vi "WriteParameter.vi"(6 "TimeOut(500)":i32=500, 9 "test":dbl[](array[numeric])=[0.0, 1.0, 111111111111111.0, 1.0, 2.0, 1.0, 1.0, 10.0, 0.0, 0.0, 0.0, 0.0, 500.0, 250.0, 2.0, 2.0, 2.0, 2.0, 0.0, 0.0, 0.0], 11 "UnitParamiterCluster":T1={"External Diameter"=0.0, "Height"=0.0, "Range"=enum."1p", "DFmin"=0.00024, "Cap_num"=0.0, "F"=0, "BIN3+"=0.0, "BIN3- "=0.0, "BIN2+"=0.0, "BIN2-"=0.0, "BIN1+"=0.0, "BIN1-"=0.0, "Frequencies"=enum."120HZ", "DFmax"=0.00024, "Part_5"=0.0, "Part_6"=0.0, "Part_4"=5.0, "Part_8"=7.0, "Part_7"=4.0, "Par_2"=4.0, "part_1"=enum."DC", "Part_9"=9.0, "Part_18"=7.0, "Part_15"=3.0, "Part_13"=2.0, "Part_14"=5.0, "Part_16"=6.0, "Internal Diameter"=0.0, "Part_14 (IR Max)"=1000000000000000.0, "SCARA Place Offset"={"Buffer"={"X"=0.0, "Y"=0.0, "Z"=0.0}, "UNLD"={"X"=0.0, "Y"=0.0, "Z"=0.0}}} {"Part_14 (IR Max)" format="%#_6p"; "Part_6" format="%#_9g"; "DFmin" format="%#_9g"; "Cap_num" format="%#_9f"; "F" items=["mF", "uF", "nF", "pF"]}) -> (0 "HiokiErrout":errorcluster, 1 "ChromaErrOut":errorcluster, 3 "TVwriteOK":bool[](array[boolean]))   [LabVIEW 2016]
uses:
  TypeDef/Enum_ErrorType.ctl
  DISGradingMachine/SubPannel/PNType/TypeDef_PNData.ctl
  DISGradingMachine/sub/MachineParType/MachineParTypeSCARA PlaceOffset.ctl
  meter global.vi
  <vilib>/Instr/_visa.llb/VISA Configure Serial Port (Instr).vi
panel:
  out "read buffer":string
  out "TV1":T3
  # "TV參數修改中,請稍候......."
  # "尺寸資訊"
  # "max 3mm  0=1mm"
  # "大於 3.56mm=0"
  # "電性測試"
  # "%"
  # "%"
  # "%"
  # "%"
  # "%"
  # "%"
  # "IR 絕緣阻抗測試"
  # "V"
  # "sec"
  # "sec"
  # "sec"
  # "GΩ"
  # "Ω"
  # "TV   耐壓測試"
  # "sec"
  # "uA"
  # "sec"
  # "KV"
  # "sec"
  # "uA"
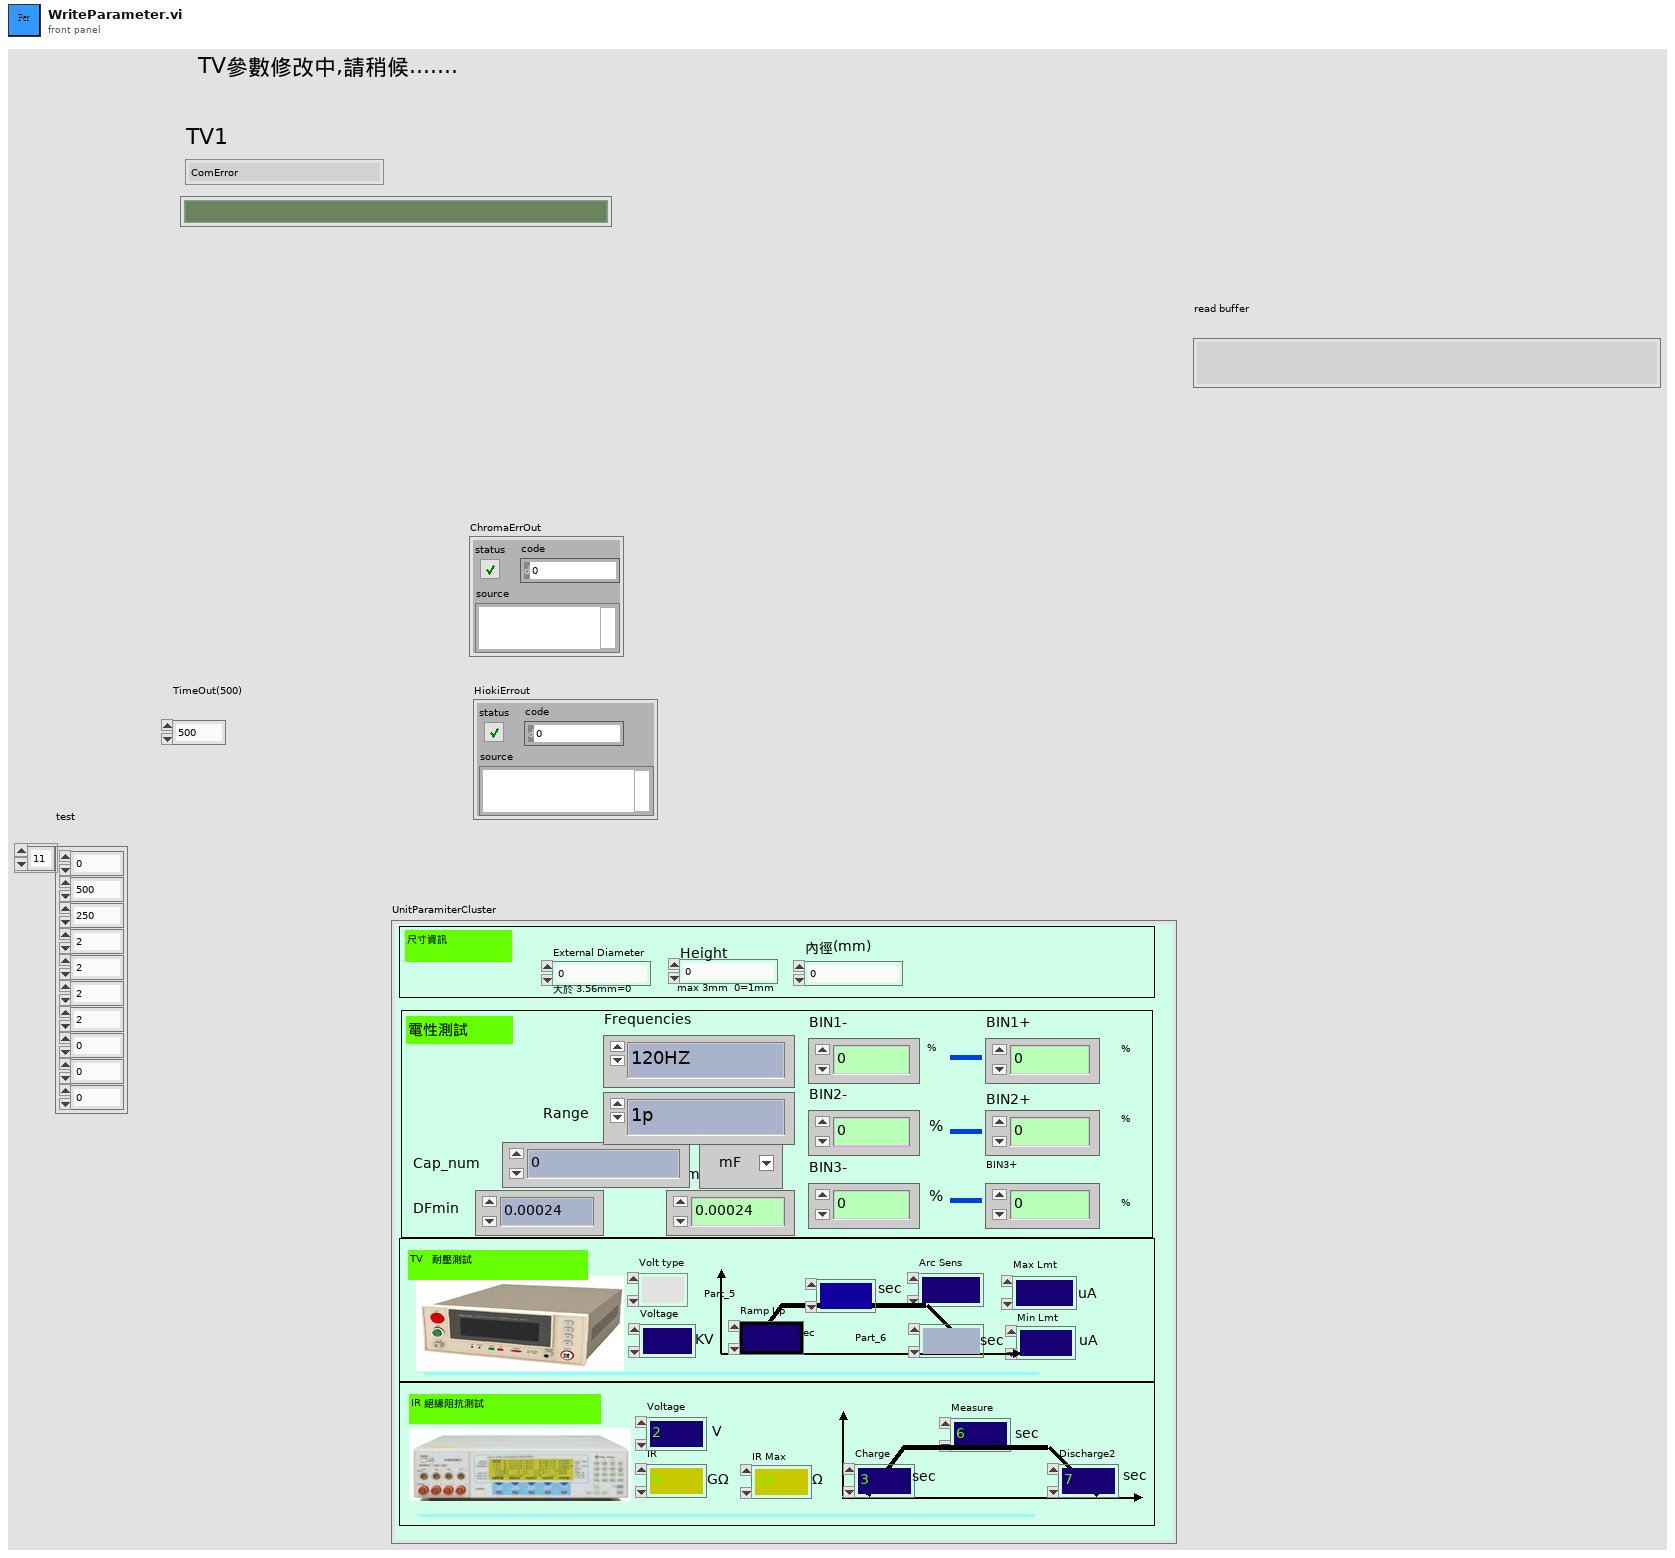
[diagram p1: front panel]
types:
  T1 = typedef "TypeDef_PNData.ctl" = cluster{"External Diameter":dbl, "Height":dbl, "Range":enum16{"1p", "2.2p", "4.7p", "10p", "22p", "47p", "100p", "220p", "470p", "1n", "2.2n", "4.7n", "10n", "22n", "47n", "100n", "220n", "470n", "1u", "2.2u", "4.7u", "10u", "22u", "47u", "100u", "220u", "470u", "1m", "AUTO", ""}, "DFmin":dbl, "Cap_num":dbl, "F":u16, "BIN3+":dbl, "BIN3- ":dbl, "BIN2+":dbl, "BIN2-":dbl, "BIN1+":dbl, "BIN1-":dbl, "Frequencies":enum16{"120HZ", "1K  HZ", "1M HZ"}, "DFmax":dbl, "Part_5":dbl, "Part_6":dbl, "Part_4":dbl, "Part_8":dbl, "Part_7":dbl, "Par_2":dbl, "part_1":enum16{"DC", "AC"}, "Part_9":dbl, "Part_18":dbl, "Part_15":dbl, "Part_13":dbl, "Part_14":dbl, "Part_16":dbl, "Internal Diameter":dbl, "Part_14 (IR Max)":dbl, "SCARA Place Offset":T2}
  T2 = typedef "MachineParTypeSCARA PlaceOffset.ctl" = cluster{"Buffer":cluster{"X":dbl, "Y":dbl, "Z":dbl}, "UNLD":cluster{"X":dbl, "Y":dbl, "Z":dbl}}
  T3 = typedef "Enum_ErrorType.ctl" = enum16{"ComError", "OK", "Command Error", "Parameter Error"}
  T4 = cluster{"Enum_mode":enum16{"AC", "DC", "IR"}, "StepIndex(1~10)":u8, "RampTime(100ms)":u16, "DwallTime(100ms)":u16, "TestTime(100ms)":u16, "Falltime(100ms)":u16, "HighLimit(100nA)":u32, "LowLimit(100nA)":u32, "ArcLimit(100nA)":u32, "InrushLimit(100nA)":u32, "Sorce(v)":u16}
  T5 = enum16{"RDT?", "IDN?", "SRT", "CBF", "SEQ?", "RMT", "SEQ", "PWS", "STP", "PWS?", "PWA", "CHS", ""}
  T6 = enum16{"RDT?", "IDN?", "SRT", "CBF", "SEQ?", "RMT", "SEQ", "PWS", "STP", "PWS?", "PWA"}
  T7 = cluster{"OFF:0/ON:1":i32, "Program Number(0~9)":i32, "DischargeTimeBeforeMeasurement":dbl, "ChargeTime":dbl, "Measuring Time":dbl, "DisCharge Time":dbl}
  T8 = cluster{"EnumFunnction":enum16{"IDN?", "test", "Stop", "Start", "Step Parameters", "Step Patameters?", "Preset Parameter", "Preset parameter?", "Offset Get/Off", "Offset?", "System Setting", "System Setting?", "KeyLock", "KeyLock?", "Initialize All Steps Parameter", "Remote/Local", "Result"}, "Hex_DA":u8, "Hex_Master":u8}
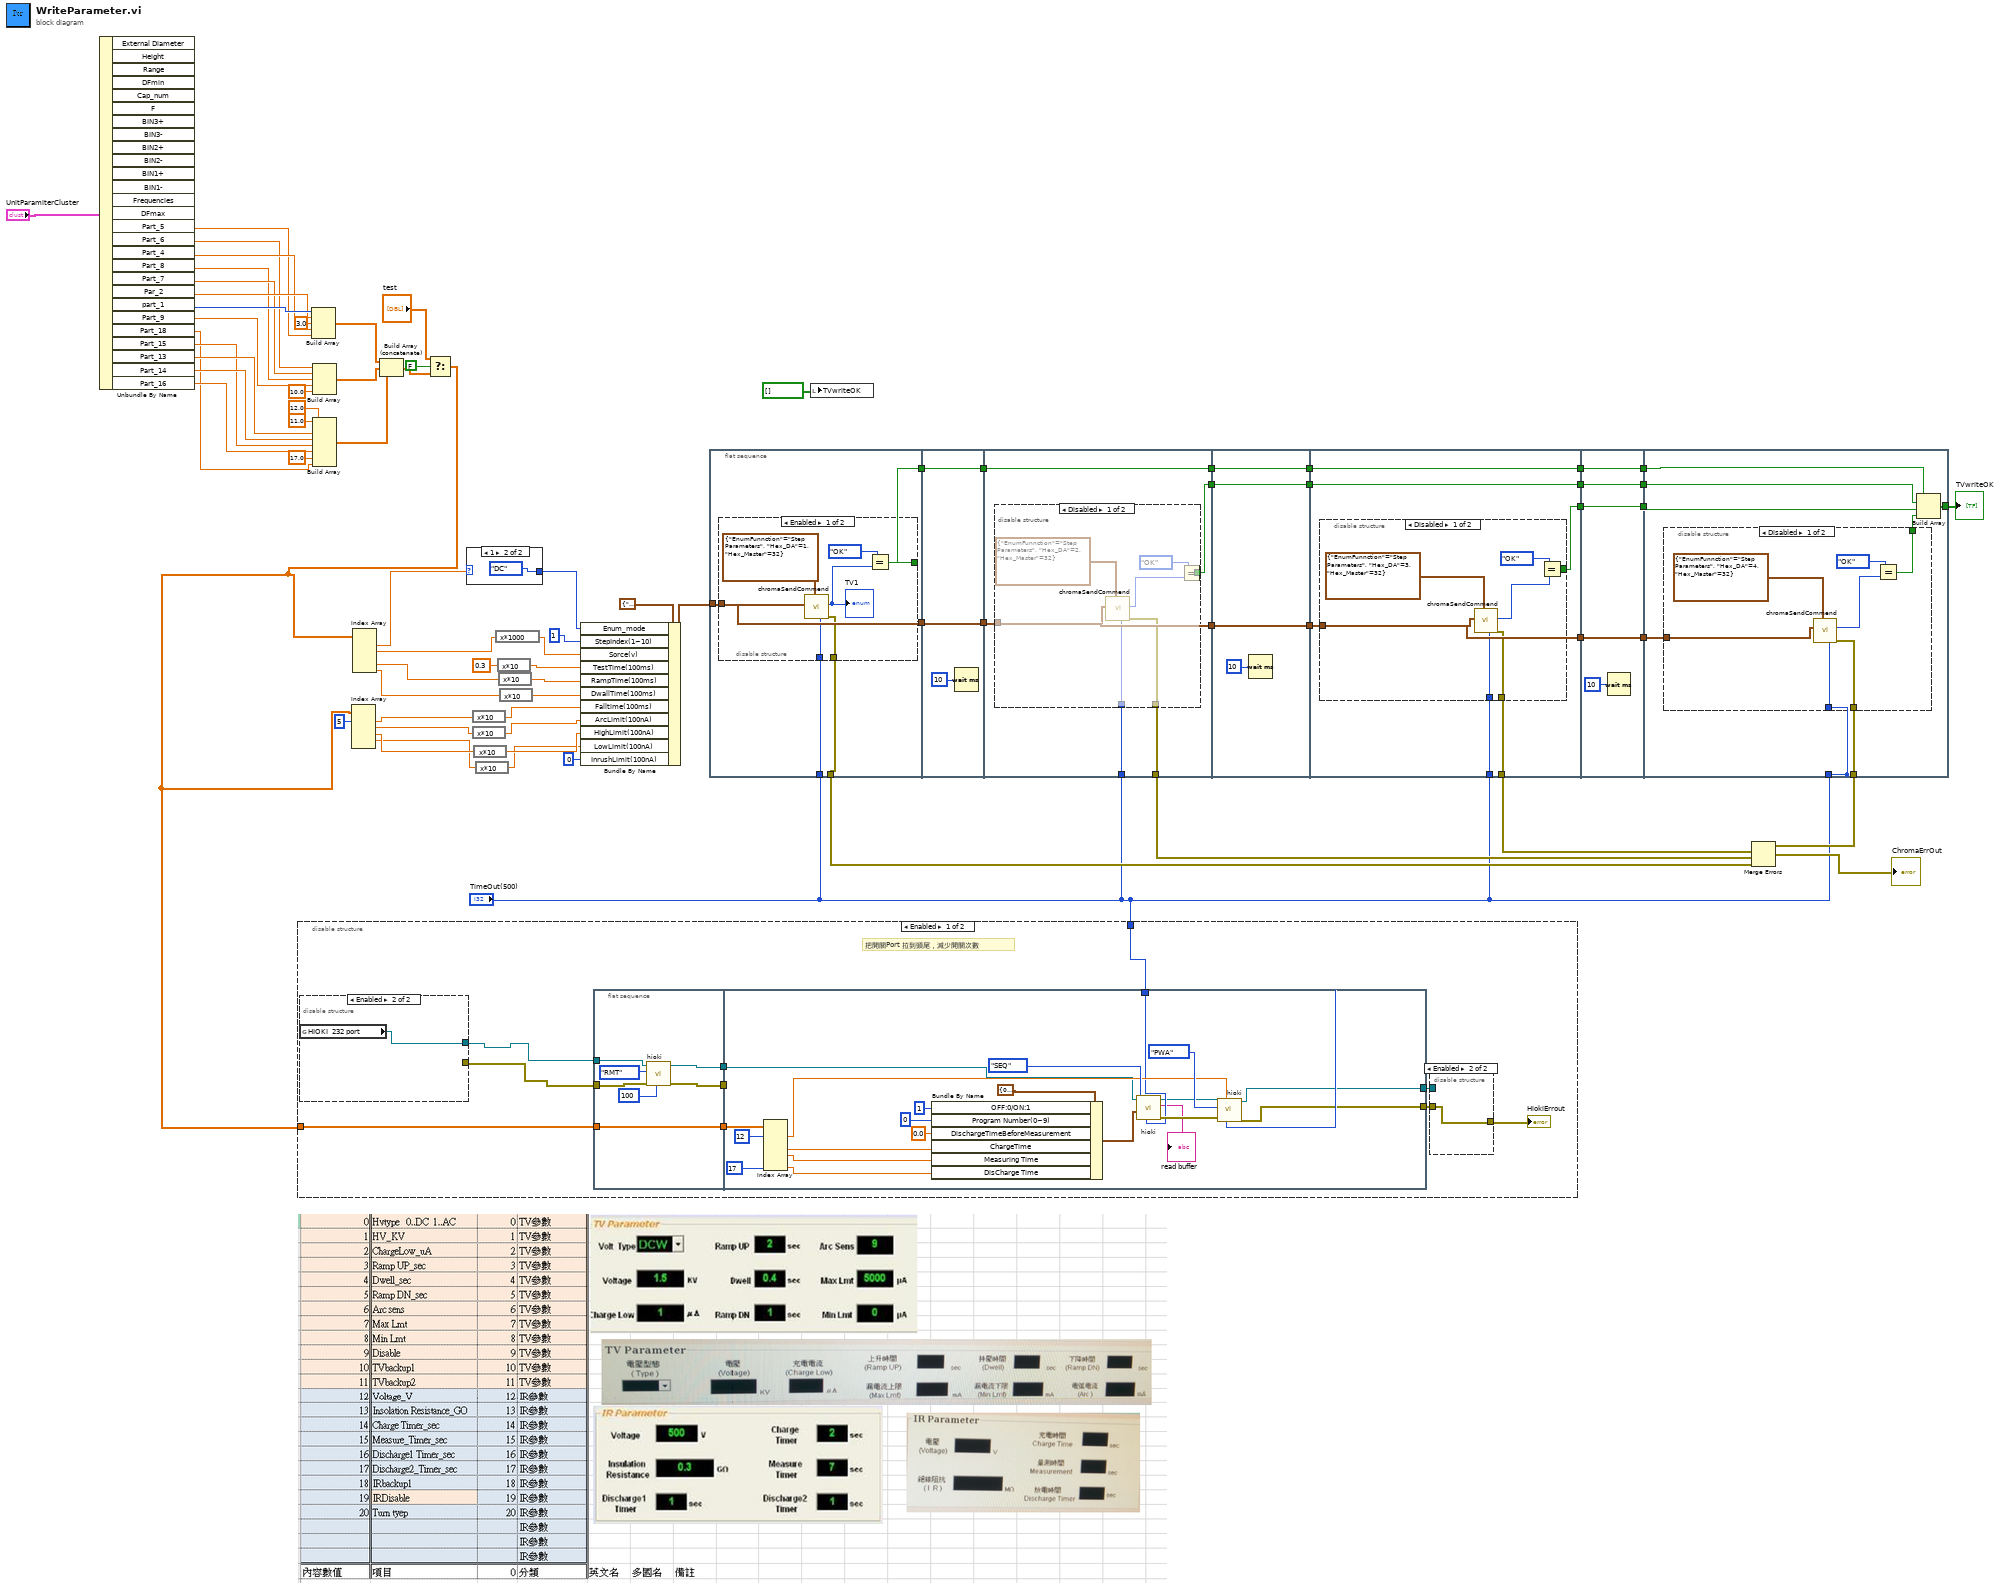
[diagram p0: block diagram]
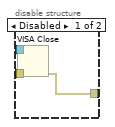
[diagram p2: hidden frame]
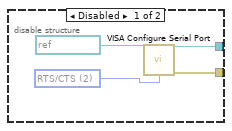
[diagram p3: hidden frame]
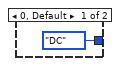
[diagram p5: hidden frame]
diagram:
  n1 = Unbundle By Name("UnitParamiterCluster") -> ("Part_5"=w21:dbl, "Part_6"=w20:dbl, "Part_4"=w22:dbl, "Part_8"=w18:dbl, "Part_7"=w19:dbl, "Par_2"=w24:dbl, "part_1"=w25:enum16{"DC", "AC"}, "Part_9"=w17:dbl, "Part_18"=w8:dbl, "Part_15"=w11:dbl, "Part_13"=w13:dbl, "Part_14"=w12:dbl, "Part_16"=w10:dbl)  [unwired: 14 out]
  n2 = Build Array(w25, w24, 3.0 ("element"), w22, w21) -> (w7:dbl[])
  n3 = Build Array(w20, w19, w18, w17, 10.0 ("element")) -> (w6:dbl[])
  n4 = Build Array(11.0 ("element"), 12.0 ("element"), w13, w12, w11, w10, 17.0 ("element"), w8) -> (w5:dbl[])
  n5 = Build Array (concatenate)(w7, w6, w5) -> (w4:dbl[])
  n6 = Select(t="test", s=FALSE, f=w4) -> (s? t:f=w1:dbl[])
  n7 = disable-structure shown="Enabled" {
    disable-tunnel: w1 -> [w82 _]
    disable-tunnel: "TimeOut(500)" -> [w81 _]
    frame Enabled {
      # "把開關Port 拉到頭尾，減少開關次數"
      n8 = disable-structure shown="Enabled" {
        disable-tunnel: [w93 _] -> w80
        disable-tunnel: [w90 w94] -> w76
        frame Disabled {
          w91 = u16 2 items=["None", "XON/XOFF", "RTS/CTS", "XON/XOFF & RTS/CTS", "DTR/DSR", "XON/XOFF & DTR/DSR"] ("flow control (0:none)")
          n9 = call-poly "VISA Configure Serial Port"("VISA resource name"=refnum<visa-resource-name> "COM3", "flow control (0:none)"=w91) -> ("VISA resource name out"=w90:refnum<visa-resource-name>, "error out"=w93:errorcluster)  [unwired: 12 in]
        }
        frame Enabled {
          n10 = global read "meter global.vi" "HIOKI  232 port"() -> (w94:refnum<visa-resource-name>)
        }
      }
      n11 = flat-sequence {
        tunnel: w82 -> [w101]
        tunnel: [w101] -> w85
        tunnel: [w98] -> w84
        tunnel: w80 -> [w97]
        tunnel: w76 -> [w95]
        tunnel: [w96] -> w83
        tunnel: w81 -> [w108]
        tunnel: w85 -> [w119]
        tunnel: w84 -> [_]
        tunnel: w83 -> [w106]
        tunnel: [w104] -> w79
        tunnel: [w103] -> w77
        frame #0 {
          n12 = call "hioki.vi"("TimeOut"=u32 100, "error in (no error)"=w97, "EnumFunction"=T5."RMT", "VISA resource name out"=w95) -> ("error out"=w98:errorcluster, "Visa_HiokiMeterOut"=w96:refnum<visa-resource-name>)  [unwired: 5 in, 1 out]
        }
        frame #1 {
          n13 = Index Array(array=w119, index #1=12 ("index"), index #6=17 ("index")) -> (element #1=w109:dbl, element #3=w116:dbl, element #4=w115:dbl, element #6=w113:dbl)  [unwired: 4 in, 2 out]
          n14 = Bundle By Name(cluster=T7 {"OFF:0/ON:1"=0, "Program Number(0~9)"=0, "DischargeTimeBeforeMeasurement"=0.0, "ChargeTime"=0.0, "Measuring Time"=0.0, "DisCharge Time"=0.0} ("Clu_SEQ"), "OFF:0/ON:1"=1, "Program Number(0~9)"=0, "DischargeTimeBeforeMeasurement"=0.0, "ChargeTime"=w116, "Measuring Time"=w115, "DisCharge Time"=w113) -> (w121:T7)
          n15 = call "hioki.vi"("TimeOut"=w108, "Clu_SEQ"=w121, "EnumFunction"=T6."SEQ", "VISA resource name out"=w106) -> ("error out"=w112:errorcluster, "read buffer"=→"read buffer":string, "Visa_HiokiMeterOut"=w105:refnum<visa-resource-name>)  [unwired: 5 in]
          n16 = call "hioki.vi"("TimeOut"=w108, "PWA(V)"=w109, "error in (no error)"=w112, "EnumFunction"=T6."PWA", "VISA resource name out"=w105) -> ("error out"=w104:errorcluster, "Visa_HiokiMeterOut"=w103:refnum<visa-resource-name>)  [unwired: 4 in, 1 out]
        }
      }
      n17 = disable-structure shown="Enabled" {
        disable-tunnel: w79 -> [w88 w89]
        disable-tunnel: [w87 w89] -> w78
        disable-tunnel: w77 -> [w86 _]
        frame Disabled {
          n18 = VISA Close(VISA resource name=w86, error in (no error)=w88) -> (error out=w87:errorcluster)
        }
        frame Enabled {
        }
      }
      "HiokiErrout" <- w78
    }
    frame Disabled {
    }
  }
  n19 = Index Array(array=w1, index #1=5 ("index")) -> (element #1=w67:dbl, element #2=w65:dbl, element #3=w63:dbl, element #4=w61:dbl)  [unwired: 4 in, 1 out]
  n20 = Index Array(array=w1) -> (element #1=w74:dbl, element #2=w46:dbl, element #4=w28:dbl, element #5=w70:dbl)  [unwired: 5 in, 1 out]
  n21 = case shown="1" w74 {
    tunnel: [enum16{"AC", "DC", "IR"}."DC" ("Enum_mode") enum16{"AC", "DC", "IR"}."DC" ("Enum_mode")] -> w73
    frame 0, Default {
    }
    frame 1 {
    }
  }
  n22 = expression code="x*10"(w67) -> (w66:dbl)
  n23 = expression code="x*10"(w65) -> (w64:dbl)
  n24 = expression code="x*10"(w63) -> (w62:dbl)
  n25 = expression code="x*10"(w61) -> (w60:dbl)
  n26 = expression code="x*1000"(w46) -> (w45:dbl)
  n27 = expression code="x*10"(0.3) -> (w29:dbl)
  n28 = expression code="x*10"(w28) -> (w71:dbl)
  n29 = expression code="x*10"(w70) -> (w69:dbl)
  n30 = Bundle By Name(cluster=T4 {"Enum_mode"=enum."AC", "StepIndex(1~10)"=1, "RampTime(100ms)"=20, "DwallTime(100ms)"=0, "TestTime(100ms)"=50, "Falltime(100ms)"=30, "HighLimit(100nA)"=10000, "LowLimit(100nA)"=1000, "ArcLimit(100nA)"=10000, "InrushLimit(100nA)"=0, "Sorce(v)"=1000} ("Clu_StepParameters"), "Enum_mode"=w73, "StepIndex(1~10)"=1, "Sorce(v)"=w45, "TestTime(100ms)"=w29, "RampTime(100ms)"=w71, "DwallTime(100ms)"=w69, "Falltime(100ms)"=w66, "ArcLimit(100nA)"=w64, "HighLimit(100nA)"=w62, "LowLimit(100nA)"=w60, "InrushLimit(100nA)"=u32 0) -> (w59:T4)
  n31 = flat-sequence {
    tunnel: w59 -> [w128]
    tunnel: [w128] -> w57
    tunnel: [w127] -> w49
    tunnel: "TimeOut(500)" -> [w126]
    tunnel: [w125] -> w39
    tunnel: [w137] -> w58
    tunnel: w57 -> [w137]
    tunnel: [w136] -> w40
    tunnel: w39 -> [w136]
    tunnel: w58 -> [w143]
    tunnel: [w143] -> w55
    tunnel: [w142] -> w50
    tunnel: "TimeOut(500)" -> [w141]
    tunnel: [w140] -> w41
    tunnel: w40 -> [w140]
    tunnel: [w139] -> w38
    tunnel: [w153] -> w56
    tunnel: w55 -> [w153]
    tunnel: [w152] -> w42
    tunnel: w41 -> [w152]
    tunnel: w38 -> [w151]
    tunnel: [w151] -> w35
    tunnel: w56 -> [w160]
    tunnel: [w160] -> w53
    tunnel: [w159] -> w51
    tunnel: "TimeOut(500)" -> [w158]
    tunnel: [w157] -> w43
    tunnel: w42 -> [w157]
    tunnel: [w156] -> w36
    tunnel: w35 -> [w156]
    tunnel: [w155] -> w33
    tunnel: [w171] -> w54
    tunnel: w53 -> [w171]
    tunnel: [w170] -> w44
    tunnel: w43 -> [w170]
    tunnel: [w169] -> w37
    tunnel: w36 -> [w169]
    tunnel: [w168] -> w34
    tunnel: w33 -> [w168]
    tunnel: w54 -> [w180]
    tunnel: [w179] -> w52
    tunnel: [w178] -> _
    tunnel: "TimeOut(500)" -> [w178]
    tunnel: w44 -> [w177]
    tunnel: w37 -> [w176]
    tunnel: w34 -> [w175]
    tunnel: [w173] -> w32
    frame #0 {
      n32 = disable-structure shown="Enabled" {
        disable-tunnel: w128 -> [w134 _]
        disable-tunnel: [w133 _] -> w127
        disable-tunnel: w126 -> [w132 _]
        disable-tunnel: [w129 _] -> w125
        frame Enabled {
          n33 = call "chromaSendCommend.vi"("Int_Port Timeout"=w132, "Clus_STDparameter"=T8 {"EnumFunnction"=enum."Step Parameters", "Hex_DA"=1, "Hex_Master"=32}, "Clu_StepParameters"=w134) -> ("ErrOut"=w133:errorcluster, "Enum_ErrorType"=w131:T3)  [unwired: 5 in, 2 out]
          "TV1" <- w131
          n34 = Equal?(x=Enum_ErrorType."OK", y=w131) -> (x = y?=w129:bool)
        }
        frame Disabled {
        }
      }
    }
    frame #1 {
      n35 = Wait (ms)(milliseconds to wait=u32 10) -> ()  [unwired: 1 out]
    }
    frame #2 {
      n36 = disable-structure shown="Disabled" {
        disable-tunnel: w143 -> [w149 _]
        disable-tunnel: [w148 _] -> w142
        disable-tunnel: w141 -> [w147 _]
        disable-tunnel: [w144 _] -> w139
        frame Disabled {
          n37 = call "chromaSendCommend.vi"("Int_Port Timeout"=w147, "Clus_STDparameter"=T8 {"EnumFunnction"=enum."Step Parameters", "Hex_DA"=2, "Hex_Master"=32}, "Clu_StepParameters"=w149) -> ("ErrOut"=w148:errorcluster, "Enum_ErrorType"=w145:T3)  [unwired: 5 in, 2 out]
          n38 = Equal?(x=Enum_ErrorType."OK", y=w145) -> (x = y?=w144:bool)
        }
        frame Enabled {
        }
      }
    }
    frame #3 {
      n39 = Wait (ms)(milliseconds to wait=u32 10) -> ()  [unwired: 1 out]
    }
    frame #4 {
      n40 = disable-structure shown="Disabled" {
        disable-tunnel: w160 -> [w166 _]
        disable-tunnel: [w165 _] -> w159
        disable-tunnel: w158 -> [w164 _]
        disable-tunnel: [w161 _] -> w155
        frame Disabled {
          (unwired) Enum_ErrorType."OK" ("x")
          n41 = call "chromaSendCommend.vi"("Int_Port Timeout"=w164, "Clus_STDparameter"=T8 {"EnumFunnction"=enum."Step Parameters", "Hex_DA"=3, "Hex_Master"=32}, "Clu_StepParameters"=w166) -> ("ErrOut"=w165:errorcluster, "Enum_ErrorType"=w162:T3)  [unwired: 5 in, 2 out]
          n42 = Equal?(x=Enum_ErrorType."OK", y=w162) -> (x = y?=w161:bool)
        }
        frame Enabled {
        }
      }
    }
    frame #5 {
      n43 = Wait (ms)(milliseconds to wait=u32 10) -> ()  [unwired: 1 out]
    }
    frame #6 {
      n44 = disable-structure shown="Disabled" {
        disable-tunnel: w180 -> [w186 _]
        disable-tunnel: [w185 _] -> w179
        disable-tunnel: w178 -> [w184 _]
        disable-tunnel: [w181 _] -> w174
        frame Disabled {
          n45 = call "chromaSendCommend.vi"("Int_Port Timeout"=w184, "Clus_STDparameter"=T8 {"EnumFunnction"=enum."Step Parameters", "Hex_DA"=4, "Hex_Master"=32}, "Clu_StepParameters"=w186) -> ("ErrOut"=w185:errorcluster, "Enum_ErrorType"=w182:T3)  [unwired: 5 in, 2 out]
          n46 = Equal?(x=Enum_ErrorType."OK", y=w182) -> (x = y?=w181:bool)
        }
        frame Enabled {
        }
      }
      n47 = Build Array(w177, w176, w175, w174) -> (w173:bool[])
    }
  }
  n48 = local write "TVwriteOK"(bool[] [] ("TVwriteOK")) -> ()
  n49 = Merge Errors(w52, w51, w50, w49) -> (→"ChromaErrOut":errorcluster)
  "TVwriteOK" <- w32
